vi "Variable Tool Setup GUI.vi"(11 "error in (no error)":errorcluster) -> (8 "OK":bool, 15 "error out":errorcluster)   [LabVIEW 2011]
uses:
  Measurments Handling/Update frequensies.ctl
  Measurments Handling/Scaling.ctl
  Measurments Handling/Alarm Setup Analog.ctl
  Measurments Handling/Alarm Responce.ctl
  Measurments Handling/Action List.ctl
  Measurments Handling/Limits.ctl
  Measurments Handling/User Setting DigitalChannel.ctl
  Measurments Handling/Alarm Responce dig.ctl
  GUI/Graph/Plot selector.ctl
  Measurments Handling/User Setting Analog Channel Bg.ctl
  Modem Status/Variable List Modem Status Digital.ctl
  Modem Status/Variable List Modem Status Analog.ctl
  Tool/Variable List Tool Digital.ctl
  Tool/Variable List Tool Analog.ctl
  Measurments Handling/Common/Variable List Common Digital.ctl
  Measurments Handling/Common/Variable List Common Analog.ctl
  emi Lib/Basic/0 - General/App/emi_Application Folder.vi
panel:
  in  "Tab Control":enum32{"Analog", "Digital / Status"}(tab)
  in  "Unit":u16(ring) items=["g"]
  in  "Calibrate":bool
  in  "User graph selection":bool
  in  "List of Analog variables":i32(listbox)
  out "Name":string
  out "Description":string
  out "Validity":T1
  in  "Scaling":T2={"Gain"=1.0, "Offset"=0.0} {"Offset" format="%.5f"; "Gain" format="%.5f"}
  in  "Limits and responses":T3={"Technical Error(NA)"={"Action"=enum."No Action", "Alarm"=FALSE}, "LL"={"Action"=enum."No Action", "Alarm"=FALSE}, "L"={"Action"=enum."No Action", "Alarm"=FALSE}, "H"={"Action"=enum."No Action", "Alarm"=FALSE}, "HH"={"Action"=enum."No Action", "Alarm"=FALSE}, "Limits"={"LL"=-inf, "L"=-inf, "H"=inf, "HH"=inf}} {"Limits"."H" format="%.3f"; "Limits"."L" format="%.3f"; "Limits"."HH" format="%.3f"; "Limits"."LL" format="%.3f"}
  in  "Upper left 1":T7 {"Line Width" items=["0", "1", "2", "3", "4", "5"]; "Var Tag" items=[""=0, "HVPSU Head Voltage(V)"=1, "HVPSU TS Voltage(V)"=2, "HVPSU Current(A)"=3, "Winch Depth(m)"=5, "Winch Line Speed(m/min)"=6, "Winch Wire Tension(kg)"=7, "Tool Max Temperature(degC)"=8, "Tool Acceleration Sum(g)"=15, "Tool Inclination(deg)"=16, "Tool Rotation(deg)"=17, "Head Voltage(V)"=27, "Stroke Extension(mm)"=38, "Stroke Force(tonne)"=41, "Stroker Upper Tension Sub(kg)"=44, "Tractor Upper Tension Sub(kg)"=48, "Tractor Lower Tension Sub(kg)"=49, "Tool (Controller) Temperature(degC)"=9, "Tool Acceleration X(g)"=12, "Tool Acceleration Y(g)"=13, "Tool Acceleration Z(g)"=14, "PSU Temp(degC)"=26, "Upper Tension Sub Temp(degC)"=30, "Tool Upper Tension Sub Raw(kg)"=31, "Lower Tension Sub Temp(degC)"=32, "Tool Lower Tension Sub Raw(kg)"=33, "Stroke In Force(tonne)"=39, "Stroke Out Force(tonne)"=40, "Stroker Pressure 1(bar)"=42, "Stroker Pressure 2(bar)"=43, "Tool Temperature sensor(degC)"=52, "Tool Motor Current(A)"=54, "TS_Signal_Quality(NA)"=58, "TS_Gain(NA)"=60, "DH_Signal_Quality(NA)"=61, "DH_Gain(NA)"=63, "Link_Status(NA)"=64, "PCP Cable Resistance(Ohm)"=4, "Tool Supply Voltage(V)"=10, "Tool (Controller) Current(A)"=11, "Tool GP Sensor 1(V)"=18, "Tool GP Sensor 2(V)"=19, "Tool (Pressure 1) Temperature(degC)"=20, "Tool Pressure 1 RAW(bar)"=21, "Tool (Pressure 2) Temperature(degC)"=22, "Tool Pressure 2 RAW(bar)"=23, "Tool (Solenoid) Temperature(degC)"=24, "Tool Solenoid Position(m)"=25, "PSU Main Voltage out(V)"=28, "PSU Main Current out(A)"=29, "Tool Motor Voltage(V)"=53, "Tool Motor Torque(tonne)"=55, "Tool weight on bit(tonne)"=56, "Tool Motor RPM(RPM)"=57, "TS_PCB_Temp(degC)"=59, "DH_PCB_Temp(degC)"=62]}
  in  "Upper left 2":T7 caption="Upper left 1" {"Line Width" items=["0", "1", "2", "3", "4", "5"]; "Var Tag" items=[""=0, "HVPSU Head Voltage(V)"=1, "HVPSU TS Voltage(V)"=2, "HVPSU Current(A)"=3, "Winch Depth(m)"=5, "Winch Line Speed(m/min)"=6, "Winch Wire Tension(kg)"=7, "Tool Max Temperature(degC)"=8, "Tool Acceleration Sum(g)"=15, "Tool Inclination(deg)"=16, "Tool Rotation(deg)"=17, "Head Voltage(V)"=27, "Stroke Extension(mm)"=38, "Stroke Force(tonne)"=41, "Stroker Upper Tension Sub(kg)"=44, "Tractor Upper Tension Sub(kg)"=48, "Tractor Lower Tension Sub(kg)"=49, "Tool (Controller) Temperature(degC)"=9, "Tool Acceleration X(g)"=12, "Tool Acceleration Y(g)"=13, "Tool Acceleration Z(g)"=14, "PSU Temp(degC)"=26, "Upper Tension Sub Temp(degC)"=30, "Tool Upper Tension Sub Raw(kg)"=31, "Lower Tension Sub Temp(degC)"=32, "Tool Lower Tension Sub Raw(kg)"=33, "Stroke In Force(tonne)"=39, "Stroke Out Force(tonne)"=40, "Stroker Pressure 1(bar)"=42, "Stroker Pressure 2(bar)"=43, "Tool Temperature sensor(degC)"=52, "Tool Motor Current(A)"=54, "TS_Signal_Quality(NA)"=58, "TS_Gain(NA)"=60, "DH_Signal_Quality(NA)"=61, "DH_Gain(NA)"=63, "Link_Status(NA)"=64, "PCP Cable Resistance(Ohm)"=4, "Tool Supply Voltage(V)"=10, "Tool (Controller) Current(A)"=11, "Tool GP Sensor 1(V)"=18, "Tool GP Sensor 2(V)"=19, "Tool (Pressure 1) Temperature(degC)"=20, "Tool Pressure 1 RAW(bar)"=21, "Tool (Pressure 2) Temperature(degC)"=22, "Tool Pressure 2 RAW(bar)"=23, "Tool (Solenoid) Temperature(degC)"=24, "Tool Solenoid Position(m)"=25, "PSU Main Voltage out(V)"=28, "PSU Main Current out(A)"=29, "Tool Motor Voltage(V)"=53, "Tool Motor Torque(tonne)"=55, "Tool weight on bit(tonne)"=56, "Tool Motor RPM(RPM)"=57, "TS_PCB_Temp(degC)"=59, "DH_PCB_Temp(degC)"=62]}
  in  "Upper right 1":T7 caption="Upper left 1" {"Line Width" items=["0", "1", "2", "3", "4", "5"]; "Var Tag" items=[""=0, "HVPSU Head Voltage(V)"=1, "HVPSU TS Voltage(V)"=2, "HVPSU Current(A)"=3, "Winch Depth(m)"=5, "Winch Line Speed(m/min)"=6, "Winch Wire Tension(kg)"=7, "Tool Max Temperature(degC)"=8, "Tool Acceleration Sum(g)"=15, "Tool Inclination(deg)"=16, "Tool Rotation(deg)"=17, "Head Voltage(V)"=27, "Stroke Extension(mm)"=38, "Stroke Force(tonne)"=41, "Stroker Upper Tension Sub(kg)"=44, "Tractor Upper Tension Sub(kg)"=48, "Tractor Lower Tension Sub(kg)"=49, "Tool (Controller) Temperature(degC)"=9, "Tool Acceleration X(g)"=12, "Tool Acceleration Y(g)"=13, "Tool Acceleration Z(g)"=14, "PSU Temp(degC)"=26, "Upper Tension Sub Temp(degC)"=30, "Tool Upper Tension Sub Raw(kg)"=31, "Lower Tension Sub Temp(degC)"=32, "Tool Lower Tension Sub Raw(kg)"=33, "Stroke In Force(tonne)"=39, "Stroke Out Force(tonne)"=40, "Stroker Pressure 1(bar)"=42, "Stroker Pressure 2(bar)"=43, "Tool Temperature sensor(degC)"=52, "Tool Motor Current(A)"=54, "TS_Signal_Quality(NA)"=58, "TS_Gain(NA)"=60, "DH_Signal_Quality(NA)"=61, "DH_Gain(NA)"=63, "Link_Status(NA)"=64, "PCP Cable Resistance(Ohm)"=4, "Tool Supply Voltage(V)"=10, "Tool (Controller) Current(A)"=11, "Tool GP Sensor 1(V)"=18, "Tool GP Sensor 2(V)"=19, "Tool (Pressure 1) Temperature(degC)"=20, "Tool Pressure 1 RAW(bar)"=21, "Tool (Pressure 2) Temperature(degC)"=22, "Tool Pressure 2 RAW(bar)"=23, "Tool (Solenoid) Temperature(degC)"=24, "Tool Solenoid Position(m)"=25, "PSU Main Voltage out(V)"=28, "PSU Main Current out(A)"=29, "Tool Motor Voltage(V)"=53, "Tool Motor Torque(tonne)"=55, "Tool weight on bit(tonne)"=56, "Tool Motor RPM(RPM)"=57, "TS_PCB_Temp(degC)"=59, "DH_PCB_Temp(degC)"=62]}
  in  "Upper right 2":T7 caption="Upper left 1" {"Line Width" items=["0", "1", "2", "3", "4", "5"]; "Var Tag" items=[""=0, "HVPSU Head Voltage(V)"=1, "HVPSU TS Voltage(V)"=2, "HVPSU Current(A)"=3, "Winch Depth(m)"=5, "Winch Line Speed(m/min)"=6, "Winch Wire Tension(kg)"=7, "Tool Max Temperature(degC)"=8, "Tool Acceleration Sum(g)"=15, "Tool Inclination(deg)"=16, "Tool Rotation(deg)"=17, "Head Voltage(V)"=27, "Stroke Extension(mm)"=38, "Stroke Force(tonne)"=41, "Stroker Upper Tension Sub(kg)"=44, "Tractor Upper Tension Sub(kg)"=48, "Tractor Lower Tension Sub(kg)"=49, "Tool (Controller) Temperature(degC)"=9, "Tool Acceleration X(g)"=12, "Tool Acceleration Y(g)"=13, "Tool Acceleration Z(g)"=14, "PSU Temp(degC)"=26, "Upper Tension Sub Temp(degC)"=30, "Tool Upper Tension Sub Raw(kg)"=31, "Lower Tension Sub Temp(degC)"=32, "Tool Lower Tension Sub Raw(kg)"=33, "Stroke In Force(tonne)"=39, "Stroke Out Force(tonne)"=40, "Stroker Pressure 1(bar)"=42, "Stroker Pressure 2(bar)"=43, "Tool Temperature sensor(degC)"=52, "Tool Motor Current(A)"=54, "TS_Signal_Quality(NA)"=58, "TS_Gain(NA)"=60, "DH_Signal_Quality(NA)"=61, "DH_Gain(NA)"=63, "Link_Status(NA)"=64, "PCP Cable Resistance(Ohm)"=4, "Tool Supply Voltage(V)"=10, "Tool (Controller) Current(A)"=11, "Tool GP Sensor 1(V)"=18, "Tool GP Sensor 2(V)"=19, "Tool (Pressure 1) Temperature(degC)"=20, "Tool Pressure 1 RAW(bar)"=21, "Tool (Pressure 2) Temperature(degC)"=22, "Tool Pressure 2 RAW(bar)"=23, "Tool (Solenoid) Temperature(degC)"=24, "Tool Solenoid Position(m)"=25, "PSU Main Voltage out(V)"=28, "PSU Main Current out(A)"=29, "Tool Motor Voltage(V)"=53, "Tool Motor Torque(tonne)"=55, "Tool weight on bit(tonne)"=56, "Tool Motor RPM(RPM)"=57, "TS_PCB_Temp(degC)"=59, "DH_PCB_Temp(degC)"=62]}
  in  "Lower left 1":T7 caption="Upper left 1" {"Line Width" items=["0", "1", "2", "3", "4", "5"]; "Var Tag" items=[""=0, "HVPSU Head Voltage(V)"=1, "HVPSU TS Voltage(V)"=2, "HVPSU Current(A)"=3, "Winch Depth(m)"=5, "Winch Line Speed(m/min)"=6, "Winch Wire Tension(kg)"=7, "Tool Max Temperature(degC)"=8, "Tool Acceleration Sum(g)"=15, "Tool Inclination(deg)"=16, "Tool Rotation(deg)"=17, "Head Voltage(V)"=27, "Stroke Extension(mm)"=38, "Stroke Force(tonne)"=41, "Stroker Upper Tension Sub(kg)"=44, "Tractor Upper Tension Sub(kg)"=48, "Tractor Lower Tension Sub(kg)"=49, "Tool (Controller) Temperature(degC)"=9, "Tool Acceleration X(g)"=12, "Tool Acceleration Y(g)"=13, "Tool Acceleration Z(g)"=14, "PSU Temp(degC)"=26, "Upper Tension Sub Temp(degC)"=30, "Tool Upper Tension Sub Raw(kg)"=31, "Lower Tension Sub Temp(degC)"=32, "Tool Lower Tension Sub Raw(kg)"=33, "Stroke In Force(tonne)"=39, "Stroke Out Force(tonne)"=40, "Stroker Pressure 1(bar)"=42, "Stroker Pressure 2(bar)"=43, "Tool Temperature sensor(degC)"=52, "Tool Motor Current(A)"=54, "TS_Signal_Quality(NA)"=58, "TS_Gain(NA)"=60, "DH_Signal_Quality(NA)"=61, "DH_Gain(NA)"=63, "Link_Status(NA)"=64, "PCP Cable Resistance(Ohm)"=4, "Tool Supply Voltage(V)"=10, "Tool (Controller) Current(A)"=11, "Tool GP Sensor 1(V)"=18, "Tool GP Sensor 2(V)"=19, "Tool (Pressure 1) Temperature(degC)"=20, "Tool Pressure 1 RAW(bar)"=21, "Tool (Pressure 2) Temperature(degC)"=22, "Tool Pressure 2 RAW(bar)"=23, "Tool (Solenoid) Temperature(degC)"=24, "Tool Solenoid Position(m)"=25, "PSU Main Voltage out(V)"=28, "PSU Main Current out(A)"=29, "Tool Motor Voltage(V)"=53, "Tool Motor Torque(tonne)"=55, "Tool weight on bit(tonne)"=56, "Tool Motor RPM(RPM)"=57, "TS_PCB_Temp(degC)"=59, "DH_PCB_Temp(degC)"=62]}
  in  "Lower left 2":T7 caption="Upper left 1" {"Line Width" items=["0", "1", "2", "3", "4", "5"]; "Var Tag" items=[""=0, "HVPSU Head Voltage(V)"=1, "HVPSU TS Voltage(V)"=2, "HVPSU Current(A)"=3, "Winch Depth(m)"=5, "Winch Line Speed(m/min)"=6, "Winch Wire Tension(kg)"=7, "Tool Max Temperature(degC)"=8, "Tool Acceleration Sum(g)"=15, "Tool Inclination(deg)"=16, "Tool Rotation(deg)"=17, "Head Voltage(V)"=27, "Stroke Extension(mm)"=38, "Stroke Force(tonne)"=41, "Stroker Upper Tension Sub(kg)"=44, "Tractor Upper Tension Sub(kg)"=48, "Tractor Lower Tension Sub(kg)"=49, "Tool (Controller) Temperature(degC)"=9, "Tool Acceleration X(g)"=12, "Tool Acceleration Y(g)"=13, "Tool Acceleration Z(g)"=14, "PSU Temp(degC)"=26, "Upper Tension Sub Temp(degC)"=30, "Tool Upper Tension Sub Raw(kg)"=31, "Lower Tension Sub Temp(degC)"=32, "Tool Lower Tension Sub Raw(kg)"=33, "Stroke In Force(tonne)"=39, "Stroke Out Force(tonne)"=40, "Stroker Pressure 1(bar)"=42, "Stroker Pressure 2(bar)"=43, "Tool Temperature sensor(degC)"=52, "Tool Motor Current(A)"=54, "TS_Signal_Quality(NA)"=58, "TS_Gain(NA)"=60, "DH_Signal_Quality(NA)"=61, "DH_Gain(NA)"=63, "Link_Status(NA)"=64, "PCP Cable Resistance(Ohm)"=4, "Tool Supply Voltage(V)"=10, "Tool (Controller) Current(A)"=11, "Tool GP Sensor 1(V)"=18, "Tool GP Sensor 2(V)"=19, "Tool (Pressure 1) Temperature(degC)"=20, "Tool Pressure 1 RAW(bar)"=21, "Tool (Pressure 2) Temperature(degC)"=22, "Tool Pressure 2 RAW(bar)"=23, "Tool (Solenoid) Temperature(degC)"=24, "Tool Solenoid Position(m)"=25, "PSU Main Voltage out(V)"=28, "PSU Main Current out(A)"=29, "Tool Motor Voltage(V)"=53, "Tool Motor Torque(tonne)"=55, "Tool weight on bit(tonne)"=56, "Tool Motor RPM(RPM)"=57, "TS_PCB_Temp(degC)"=59, "DH_PCB_Temp(degC)"=62]}
  in  "Lower right 1":T7 caption="Upper left 1" {"Line Width" items=["0", "1", "2", "3", "4", "5"]; "Var Tag" items=[""=0, "HVPSU Head Voltage(V)"=1, "HVPSU TS Voltage(V)"=2, "HVPSU Current(A)"=3, "Winch Depth(m)"=5, "Winch Line Speed(m/min)"=6, "Winch Wire Tension(kg)"=7, "Tool Max Temperature(degC)"=8, "Tool Acceleration Sum(g)"=15, "Tool Inclination(deg)"=16, "Tool Rotation(deg)"=17, "Head Voltage(V)"=27, "Stroke Extension(mm)"=38, "Stroke Force(tonne)"=41, "Stroker Upper Tension Sub(kg)"=44, "Tractor Upper Tension Sub(kg)"=48, "Tractor Lower Tension Sub(kg)"=49, "Tool (Controller) Temperature(degC)"=9, "Tool Acceleration X(g)"=12, "Tool Acceleration Y(g)"=13, "Tool Acceleration Z(g)"=14, "PSU Temp(degC)"=26, "Upper Tension Sub Temp(degC)"=30, "Tool Upper Tension Sub Raw(kg)"=31, "Lower Tension Sub Temp(degC)"=32, "Tool Lower Tension Sub Raw(kg)"=33, "Stroke In Force(tonne)"=39, "Stroke Out Force(tonne)"=40, "Stroker Pressure 1(bar)"=42, "Stroker Pressure 2(bar)"=43, "Tool Temperature sensor(degC)"=52, "Tool Motor Current(A)"=54, "TS_Signal_Quality(NA)"=58, "TS_Gain(NA)"=60, "DH_Signal_Quality(NA)"=61, "DH_Gain(NA)"=63, "Link_Status(NA)"=64, "PCP Cable Resistance(Ohm)"=4, "Tool Supply Voltage(V)"=10, "Tool (Controller) Current(A)"=11, "Tool GP Sensor 1(V)"=18, "Tool GP Sensor 2(V)"=19, "Tool (Pressure 1) Temperature(degC)"=20, "Tool Pressure 1 RAW(bar)"=21, "Tool (Pressure 2) Temperature(degC)"=22, "Tool Pressure 2 RAW(bar)"=23, "Tool (Solenoid) Temperature(degC)"=24, "Tool Solenoid Position(m)"=25, "PSU Main Voltage out(V)"=28, "PSU Main Current out(A)"=29, "Tool Motor Voltage(V)"=53, "Tool Motor Torque(tonne)"=55, "Tool weight on bit(tonne)"=56, "Tool Motor RPM(RPM)"=57, "TS_PCB_Temp(degC)"=59, "DH_PCB_Temp(degC)"=62]}
  in  "Lower right 2":T7 caption="Upper left 1" {"Line Width" items=["0", "1", "2", "3", "4", "5"]; "Var Tag" items=[""=0, "HVPSU Head Voltage(V)"=1, "HVPSU TS Voltage(V)"=2, "HVPSU Current(A)"=3, "Winch Depth(m)"=5, "Winch Line Speed(m/min)"=6, "Winch Wire Tension(kg)"=7, "Tool Max Temperature(degC)"=8, "Tool Acceleration Sum(g)"=15, "Tool Inclination(deg)"=16, "Tool Rotation(deg)"=17, "Head Voltage(V)"=27, "Stroke Extension(mm)"=38, "Stroke Force(tonne)"=41, "Stroker Upper Tension Sub(kg)"=44, "Tractor Upper Tension Sub(kg)"=48, "Tractor Lower Tension Sub(kg)"=49, "Tool (Controller) Temperature(degC)"=9, "Tool Acceleration X(g)"=12, "Tool Acceleration Y(g)"=13, "Tool Acceleration Z(g)"=14, "PSU Temp(degC)"=26, "Upper Tension Sub Temp(degC)"=30, "Tool Upper Tension Sub Raw(kg)"=31, "Lower Tension Sub Temp(degC)"=32, "Tool Lower Tension Sub Raw(kg)"=33, "Stroke In Force(tonne)"=39, "Stroke Out Force(tonne)"=40, "Stroker Pressure 1(bar)"=42, "Stroker Pressure 2(bar)"=43, "Tool Temperature sensor(degC)"=52, "Tool Motor Current(A)"=54, "TS_Signal_Quality(NA)"=58, "TS_Gain(NA)"=60, "DH_Signal_Quality(NA)"=61, "DH_Gain(NA)"=63, "Link_Status(NA)"=64, "PCP Cable Resistance(Ohm)"=4, "Tool Supply Voltage(V)"=10, "Tool (Controller) Current(A)"=11, "Tool GP Sensor 1(V)"=18, "Tool GP Sensor 2(V)"=19, "Tool (Pressure 1) Temperature(degC)"=20, "Tool Pressure 1 RAW(bar)"=21, "Tool (Pressure 2) Temperature(degC)"=22, "Tool Pressure 2 RAW(bar)"=23, "Tool (Solenoid) Temperature(degC)"=24, "Tool Solenoid Position(m)"=25, "PSU Main Voltage out(V)"=28, "PSU Main Current out(A)"=29, "Tool Motor Voltage(V)"=53, "Tool Motor Torque(tonne)"=55, "Tool weight on bit(tonne)"=56, "Tool Motor RPM(RPM)"=57, "TS_PCB_Temp(degC)"=59, "DH_PCB_Temp(degC)"=62]}
  out "Name Dig":string
  out "NA Indicatino":string caption="NA"
  out "Description Dig":string caption="Description"
  out "Validity Dig":T1 caption="Validity"
  out "On indication":string caption="ON / TRUE"
  out "Off Indication":string caption="OFF / FALSE"
  in  "User settings":T8
  in  "List of Digital variables":i32(listbox)
  out "Mode":bool
  in  "Help":bool
  in  "Cancel":bool
  in  "OK":bool
  # "Tab header s can be changed as wanted\n\nCustom can be used for completly ccutom behavior,\nmust then highjack  an other hidden page, for settings"
  # "Add custom behavior taht cvan not be replicated by a simple cluster with valisdity checking"
  # "Information"
  # "Usage"
  # "Chart default IO channels"
  # "Information"
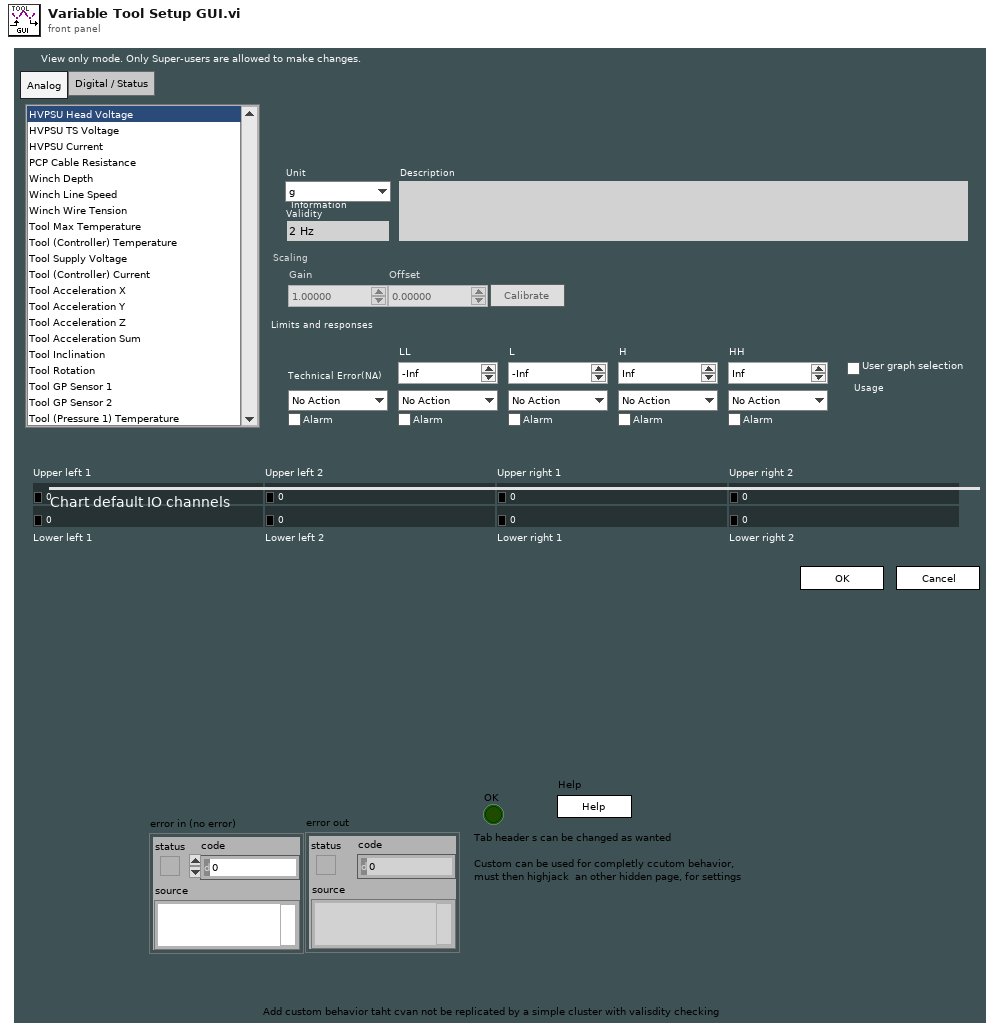
[diagram p1: front panel]
types:
  T1 = typedef "Update frequensies.ctl" = enum16{"2 Hz", "1 Hz", "0.1 Hz"}
  T2 = typedef "Scaling.ctl" = cluster{"Gain":dbl, "Offset":dbl}
  T3 = typedef "Alarm Setup Analog.ctl" = cluster{"Technical Error(NA)":T4, "LL":T4, "L":T4, "H":T4, "HH":T4, "Limits":T6}
  T4 = typedef "Alarm Responce.ctl" = cluster{"Action":T5, "Alarm":bool}
  T5 = typedef "Action List.ctl" = enum16{"No Action", "Stop Motor", "Turn Off HV"}
  T6 = typedef "Limits.ctl" = cluster{"LL":dbl, "L":dbl, "H":dbl, "HH":dbl}
  T7 = typedef "Plot selector.ctl" = cluster{"Var Tag":u16, "Color":u32, "Line Width":u16}
  T8 = typedef "User Setting DigitalChannel.ctl" = cluster{"Responses":cluster{"Technical Error (NA)":T4, "OFF / FALSE":T9, "ON / TRUE":T9}}
  T9 = typedef "Alarm Responce dig.ctl" = cluster{"Action":T5, "Alarm":bool, "Exclamation":bool}
  T10 = enum16{"GET", "SET", "Get from Ini", "Put in Ini"}
  T11 = typedef "User Indikator.ctl" = cluster{"User Name":string, "Super User":T12}
  T12 = typedef "Super User bool indikator.ctl" = bool
  T13 = enum8{"Enabled", "Disabled", "Disabled and Grayed Out"}
  T14 = typedef "Graph default cluseter.ctl" = cluster{"UL1":T7, "UL2":T7, "UR1":T7, "UR2":T7, "LL1":T7, "LL2":T7, "LR1":T7, "LR2":T7}
  T15 = typedef "Fixed Analog Channel Definition.ctl" = cluster{"ID":u16, "Name":string, "Quantity":T16, "Unit":string, "Maximum upd":T1, "Comment":string, "Help file Name":string, "Help file Section ":string, "Category":T17, "User adjustable Scaling":bool, "Default Scaling":T2, "Default Unit":i32, "Classification":T18}
  T16 = typedef "Quantity enum.ctl" = enum16{"NA", "Acceleration", "Angle", "Current", "Force", "Distance", "Pressure", "Resistance", "Rotational Speed", "Speed", "Temperature", "Tension", "Torque", "Voltage", "Weight"}
  T17 = typedef "Channel catagory Enum.ctl" = enum16{"No Category", "Power", "Temperature", "Pressure"}
  T18 = typedef "Channel Classification Enum.ctl" = enum16{"Basic", "Advanced", "Expert", "Unused"}
  T19 = typedef "Fixed Digital Channel Definition.ctl" = cluster{"ID":u16, "Name":string, "NA Text":string, "Off Text":string, "On Text":string, "Maximum upd":T1, "Comment":string, "Help file Name":string, "Help file Section ":string, "Catagory":T17, "In use":bool}
  T20 = typedef "User Setting Analog Channel Bg.ctl" = cluster{"Scaling":T2, "Limits and responces":T3, "Allow Graph selection by user":bool, "Unit":u16}
  T21 = typedef "Variable List Modem Status Digital.ctl" = enum16{"TMU_LINK_STATUS"}
  T22 = typedef "Variable List Modem Status Analog.ctl" = enum16{"TS_Signal_Quality", "TS_PCB_Temp", "TS_Gain", "DH_Signal_Quality", "DH_PCB_Temp", "DH_Gain", "Link_Status"}
  T23 = typedef "Variable List Tool Digital.ctl" = enum16{"Tool Error Controller", "Tool Stopped Controller", "Tool Relay 1", "Tool Relay 2", "Tool Both Relays", "Tool node Pressure 1", "Tool Error Pressure 1", "Tool Stopped Pressure 1", "Tool node Pressure 2", "Tool Error Pressure 2", "Tool Stopped Pressure 2", "Tool node Solenoid", "Tool Error Solenoid", "Tool Stopped Solenoid", "Tool Solenoid 1", "Tool Solenoid 2", "Tool Solenoid 3", "Tool node PSU", "Tool Error PSU", "Tool Stopped PSU", "Upper Tension Sub", "Tool Error Upper Tension Sub", "Tool Stopped Upper Tension Sub", "Lower Tension Sub", "Tool Error Lower Tension Sub", "Tool Stopped Lower Tension Sub", "Stroke Target seeking", "Stroke Moving Out", "Stroke Moving Inn", "Stroke valves set for Out", "Stroke valves set for In", "Stroke In (force)", "Stroke Out (force)", "Stroke Force decreasing(in)", "Stroke Force decreasing(out)", "Stroke Force change not correct", "Stroke SLIPS established P1", "Stroke SLIPS established P2", "Stroke SLIPS established", "Stroke Pressure Monitor Ongoing", "Stroke Pressure Monitor Ending ", "Tool Stroke enable Valve", "Tool Stroke direction Valve", "Tool Anchor Valve", "Stroker Var19 - Reserved", "Stroker Var20 - Reserved", "Stroker Var21 - Reserved", "Stroker Var22 - Reserved", "Stroker Var23 - Reserved", "Stroker Var24 - Reserved", "Tractor Var1 - Reserved", "Tractor Var2 - Reserved", "Tractor Var3 - Reserved", "Tractor Var4 - Reserved", "Tractor Var5 - Reserved", "Tractor Var6 - Reserved", "Tractor Var7 - Reserved", "Tractor Var8 - Reserved", "Oil filling mode", "Mill Bit Direction", "Position control", "Anchor", "Driller Var5 - Reserved", "Driller Var6 - Reserved", "Driller Var7 - Reserved", "Driller Var8 - Reserved"}
  T24 = typedef "Variable List Tool Analog.ctl" = enum16{"Tool Max Temperature", "Tool (Controller) Temperature", "Tool Supply Voltage", "Tool (Controller) Current", "Tool Acceleration X", "Tool Acceleration Y", "Tool Acceleration Z", "Tool Acceleration Sum", "Tool Inclination", "Tool Rotation", "Tool GP Sensor 1", "Tool GP Sensor 2", "Tool (Pressure 1) Temperature", "Tool Pressure 1 RAW", "Tool (Pressure 2) Temperature", "Tool Pressure 2 RAW", "Tool (Solenoid) Temperature", "Tool Solenoid Position", "PSU Temp", "Head Voltage", "PSU Main Voltage out", "PSU Main Current out", "Upper Tension Sub Temp", "Tool Upper Tension Sub Raw", "Lower Tension Sub Temp", "Tool Lower Tension Sub Raw", "Tool Var27 - Reserved", "Tool Var28 - Reserved", "Tool Var29 - Reserved", "Tool Var30 - Reserved", "Stroke Extension", "Stroke In Force", "Stroke Out Force", "Stroke Force", "Stroker Pressure 1", "Stroker Pressure 2", "Stroker Upper Tension Sub", "Stroker Lower Tension Sub", "Stroker Var09 - Reserved", "Stroker Var10 - Reserved", "Tractor Upper Tension Sub", "Tractor Lower Tension Sub", "Tractor Var03 - Reserved", "Tractor Var04 - Reserved", "Tool Temperature sensor", "Tool Motor Voltage", "Tool Motor Current", "Tool Motor Torque", "Tool weight on bit", "Tool Motor RPM"}
  T25 = typedef "Variable List Common Digital.ctl" = enum16{"PCP Connected", "PCP PC Control", "HV PSU connected", "HV PSU HV Active", "Modem Connected", "Tool Connected", "CanBus interface"}
  T26 = typedef "Variable List Common Analog.ctl" = enum16{"HVPSU Head Voltage", "HVPSU TS Voltage", "HVPSU Current", "PCP Cable Resistance", "Winch Depth", "Winch Line Speed", "Winch Wire Tension"}
  T27 = cluster{"Keep":bool, "Zero":bool, "2 point":bool}
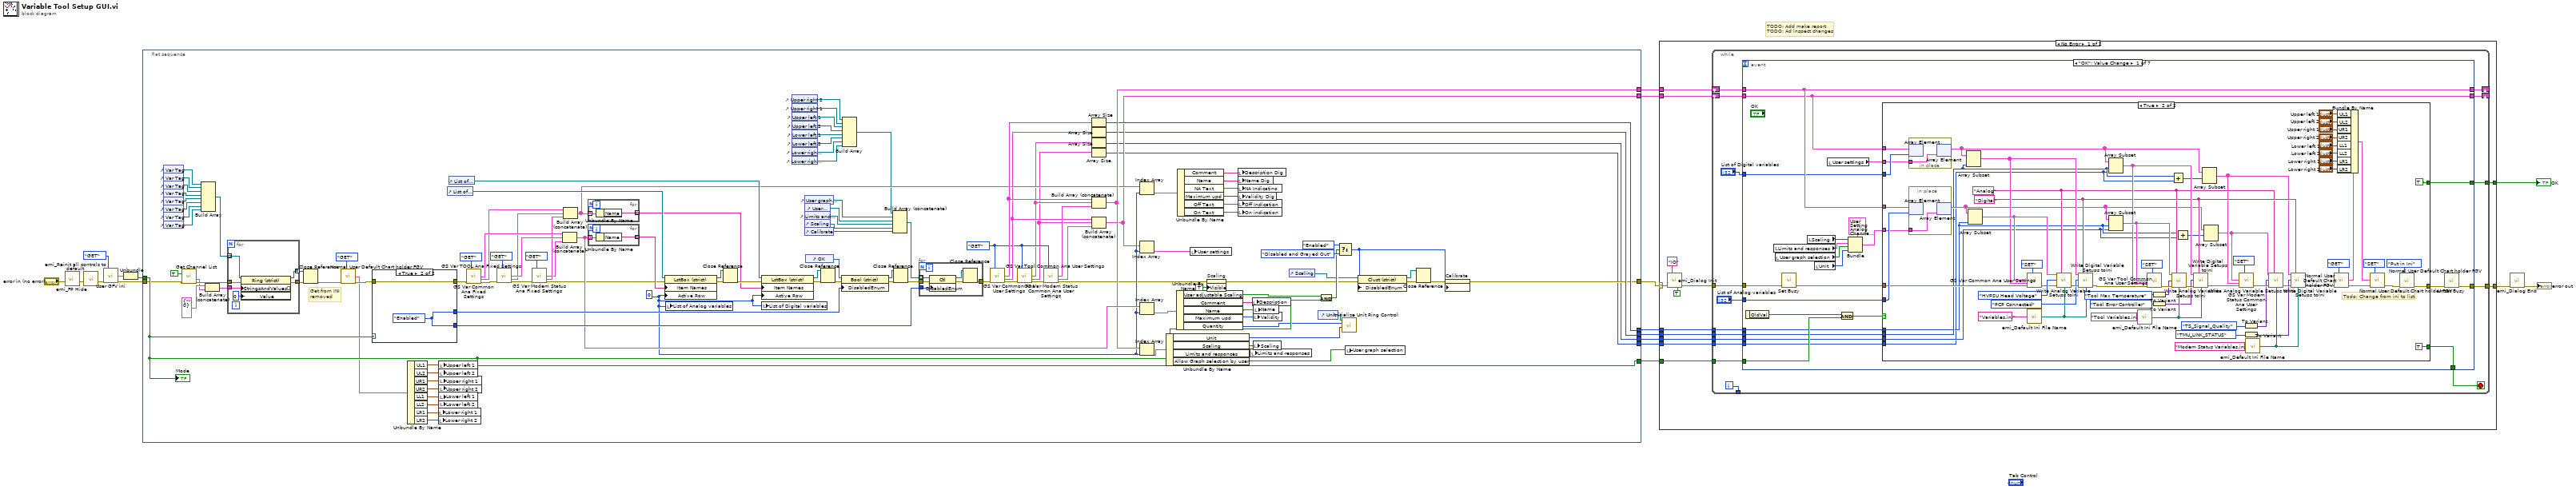
[diagram p0: block diagram]
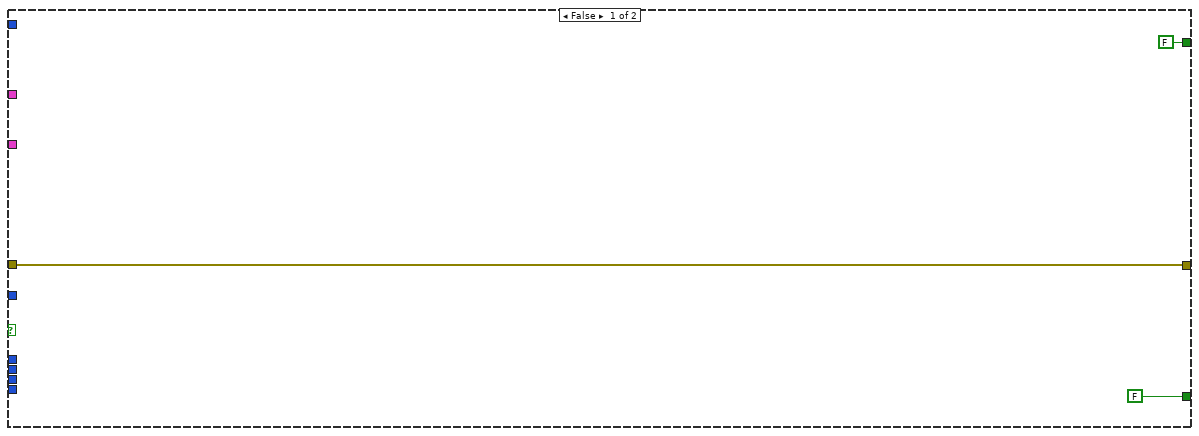
[diagram p2: hidden frame]
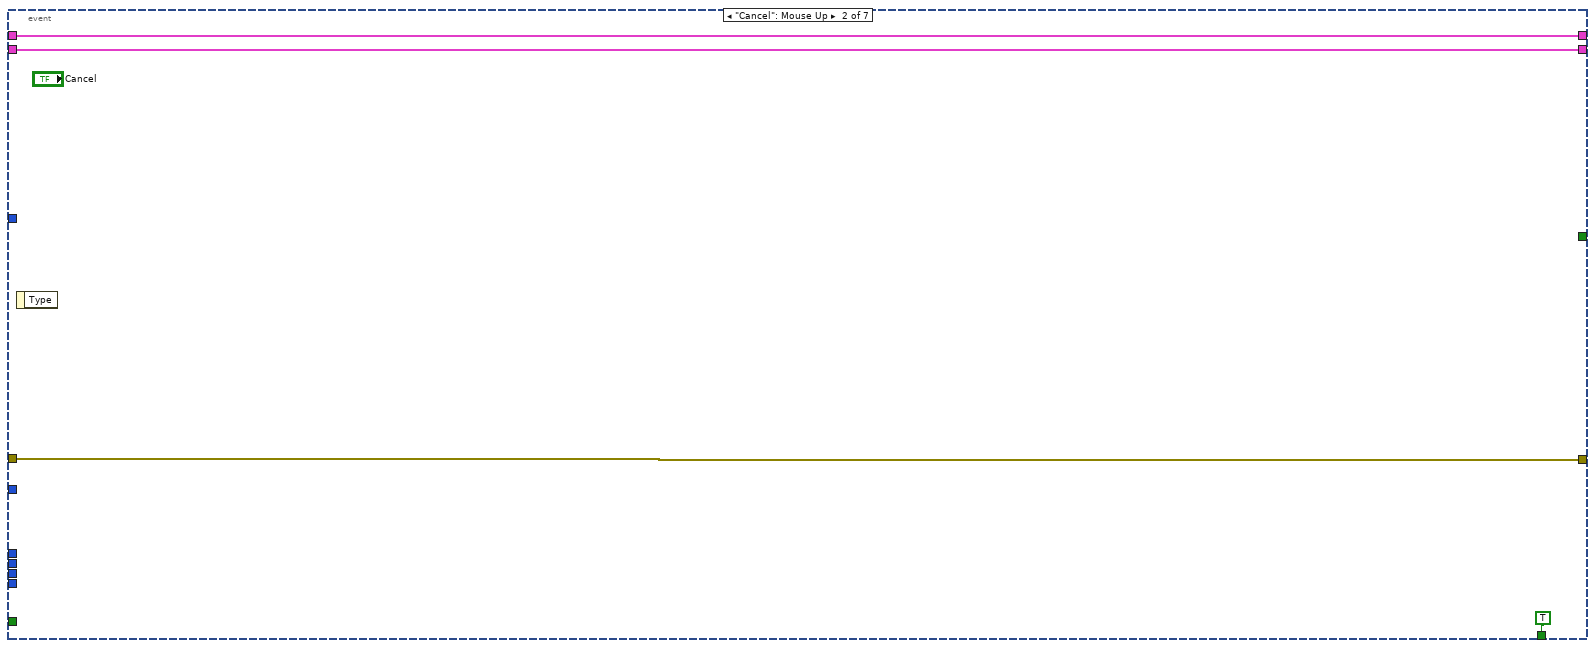
[diagram p3: hidden frame]
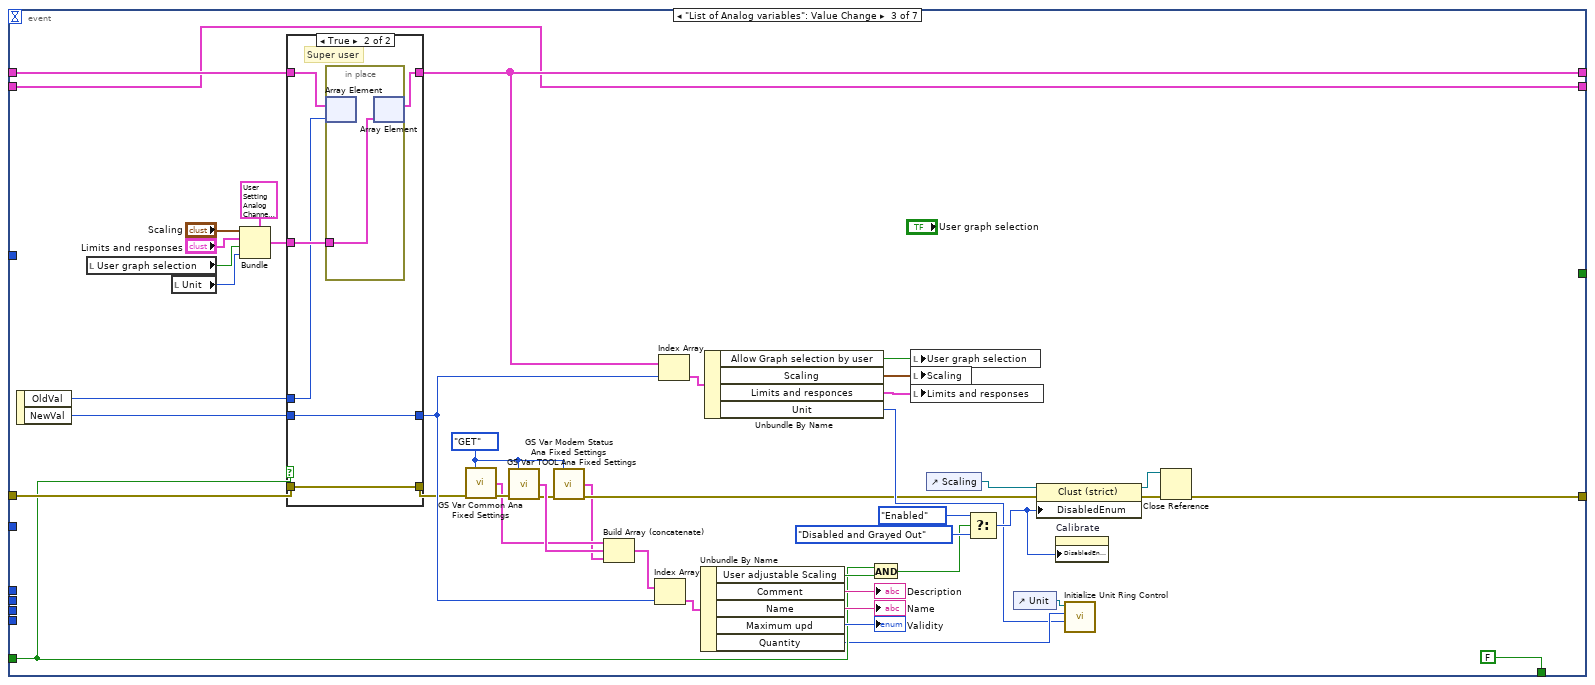
[diagram p4: hidden frame]
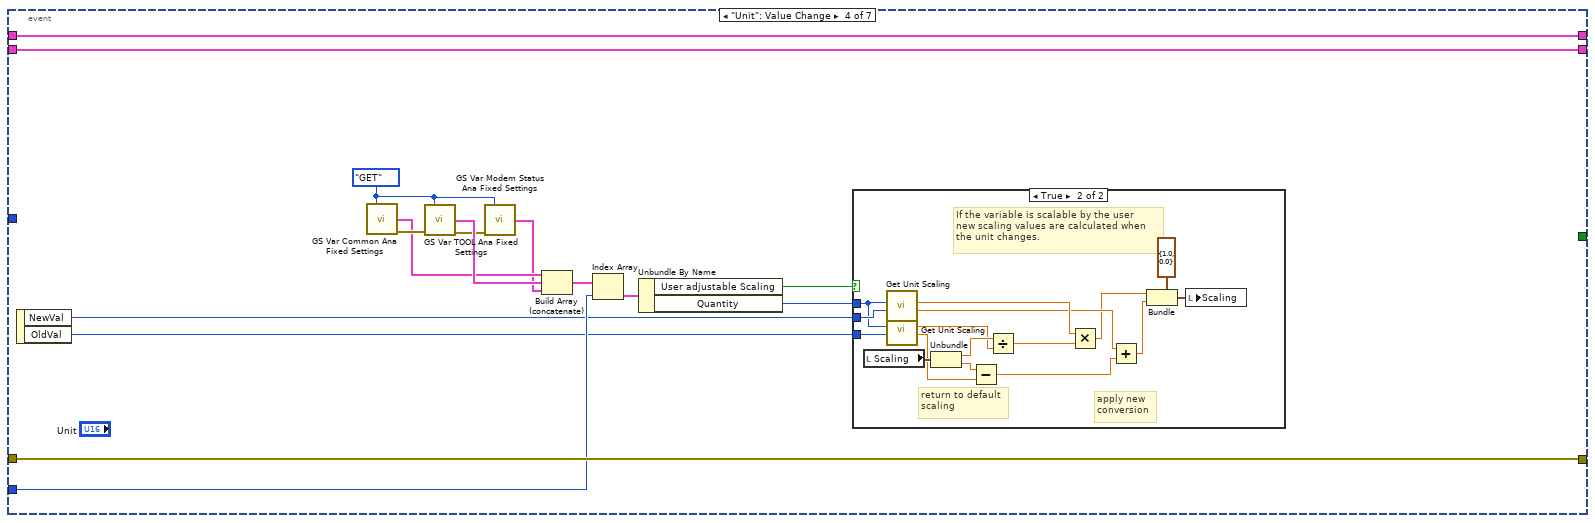
[diagram p6: hidden frame]
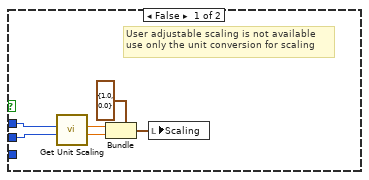
[diagram p7: hidden frame]
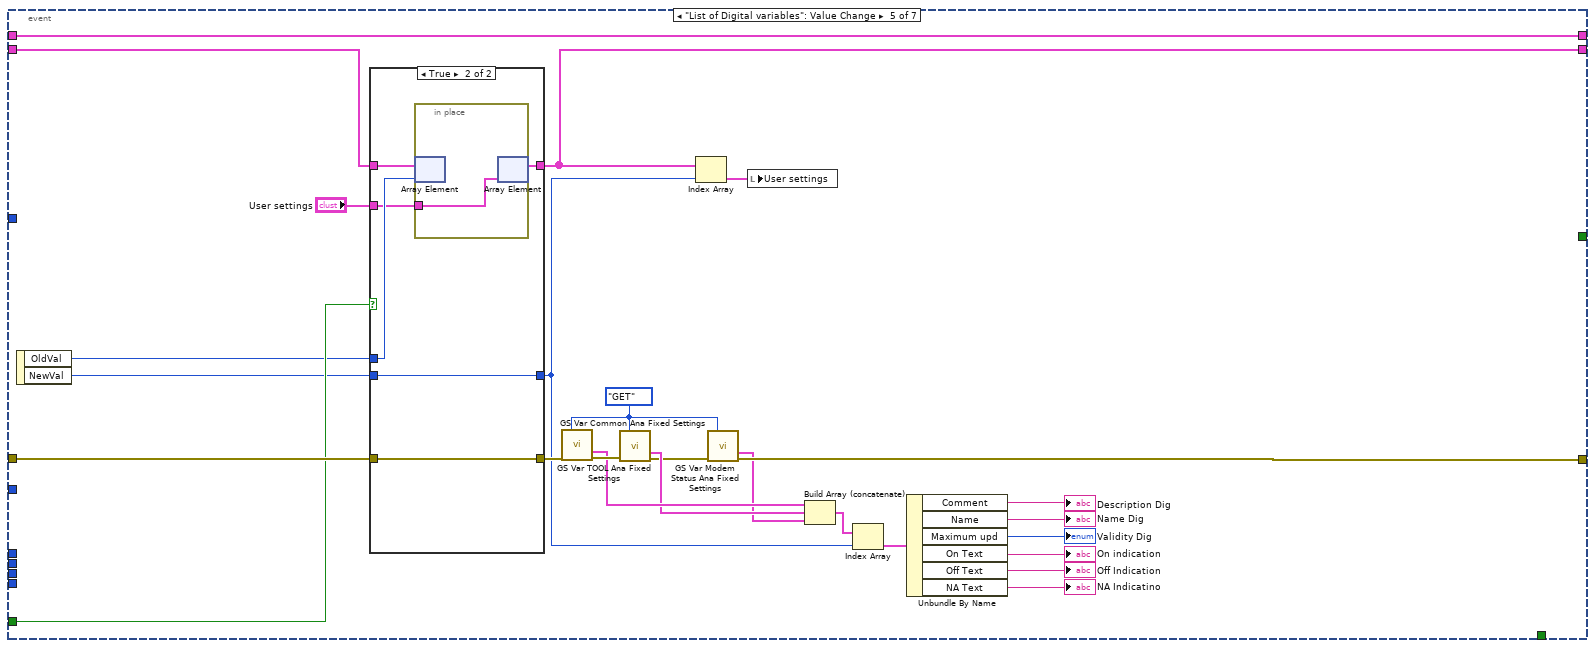
[diagram p8: hidden frame]
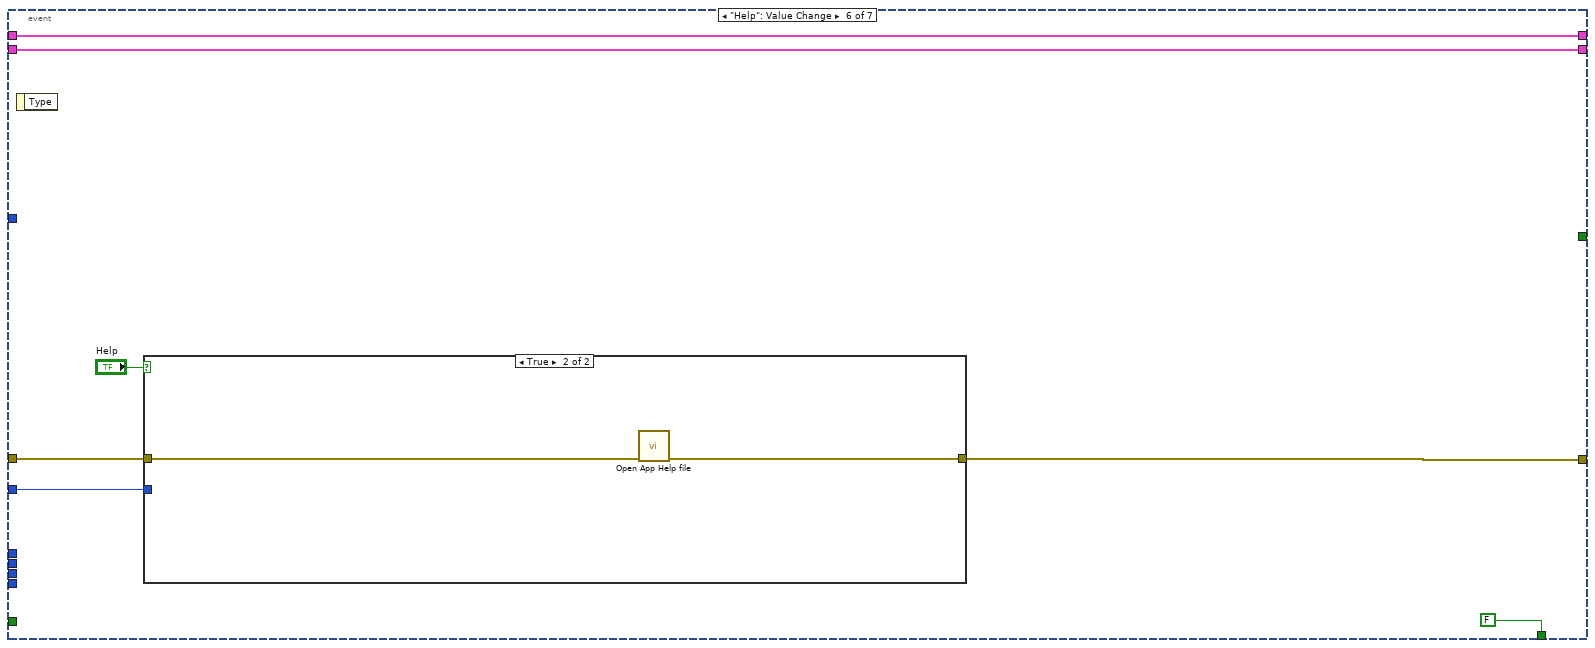
[diagram p10: hidden frame]
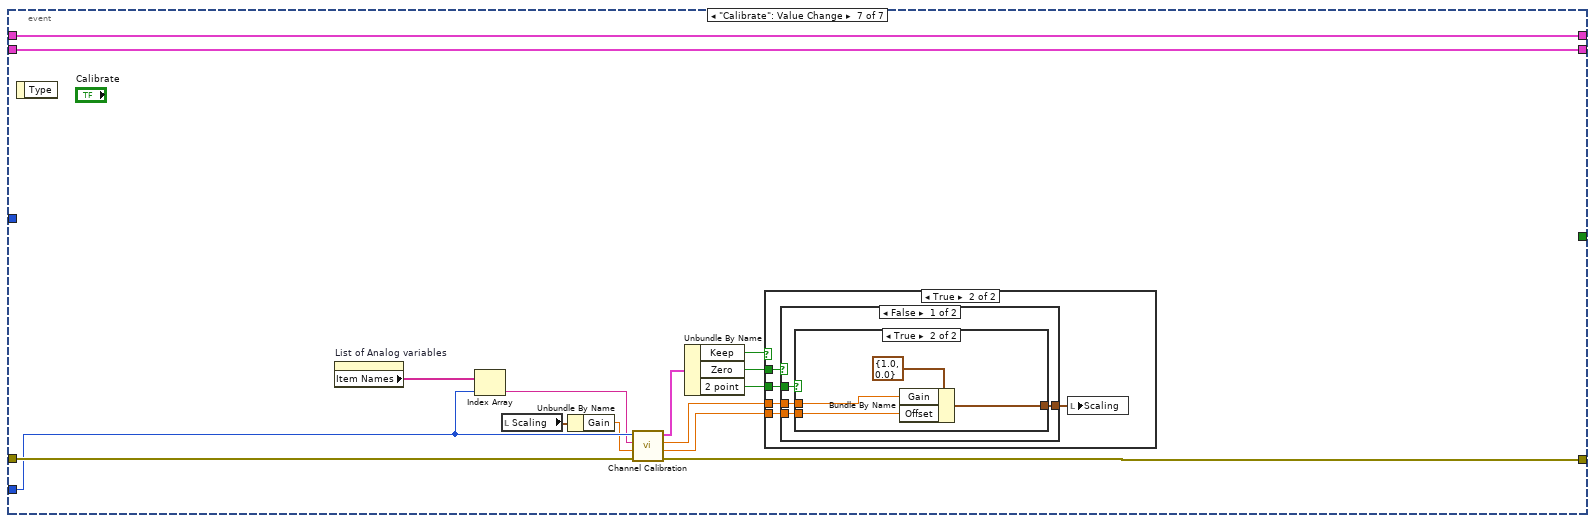
[diagram p12: hidden frame]
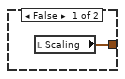
[diagram p14: hidden frame]
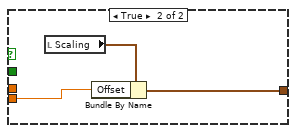
[diagram p15: hidden frame]
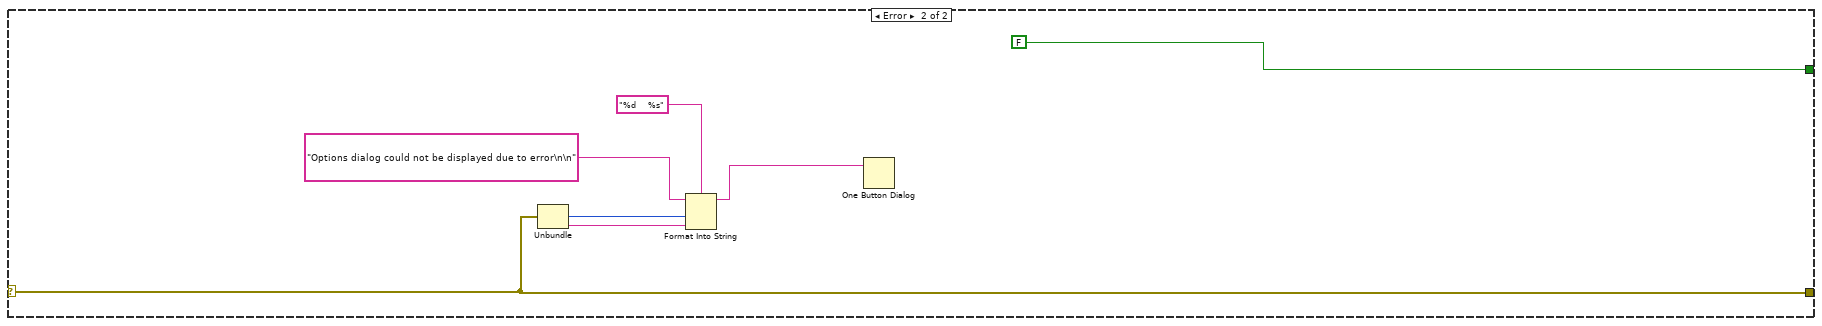
[diagram p16: hidden frame]
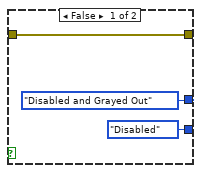
[diagram p17: hidden frame]
diagram:
  # "TODO: Add make report\nTODO: Ad inspect changes"
  n1 = call "emi_FP Hide.vi"("error in (no error)"="error in (no error)") -> ("error out"=w14:errorcluster)  [unwired: 13 in, 1 out]
  n2 = call "emi_Reinit all controls to default.vi"("error in (no error)"=w14) -> ("error out"=w12:errorcluster)  [unwired: 13 in, 1 out]
  n3 = call "User GFV ini.vi"("Action(GET)"=T10."GET", "error in (no error)"=w12) -> ("User ID out"=w11:T11, "error out"=w10:errorcluster)  [unwired: 12 in]
  n4 = Unbundle(w11) -> ("Super User"=w9:T12)  [unwired: 1 out]
  n5 = flat-sequence {
    tunnel: [w45] -> w13
    tunnel: w10 -> [w61]
    tunnel: w9 -> [w87]
    tunnel: [w87] -> w8
    tunnel: [w124] -> w7
    tunnel: [w122] -> w5
    tunnel: [w91] -> w4
    tunnel: [w90] -> w3
    tunnel: [w21] -> w2
    tunnel: [w20] -> w1
    frame #0 {
      w26 = enum16{"GET", "SET"}."GET" ("Action(GET)")
      w93 = 0 ("Active Row:Active Row Number")
      # "Get from INI\nremoved"
      n6 = control-ref of="Var Tag"() -> (w78:refnum<vi>)
      n7 = control-ref of="Var Tag"() -> (w79:refnum<vi>)
      n8 = control-ref of="Var Tag"() -> (w80:refnum<vi>)
      n9 = control-ref of="Var Tag"() -> (w81:refnum<vi>)
      n10 = control-ref of="Var Tag"() -> (w82:refnum<vi>)
      n11 = control-ref of="Var Tag"() -> (w83:refnum<vi>)
      n12 = control-ref of="Var Tag"() -> (w84:refnum<vi>)
      n13 = control-ref of="Var Tag"() -> (w85:refnum<vi>)
      n14 = call "Get Channel List.vi"("Force all(F)"=TRUE, "error in"=w61) -> ("Ring list"=w71:cluster{"String":string, "Value":u16}[], "error out"=w76:errorcluster)  [unwired: 9 in, 3 out]
      n15 = Build Array(w78, w79, w80, w81, w82, w83, w84, w85) -> (w86:refnum<vi>[])
      n16 = Build Array (concatenate)(cluster{"String":string, "Value":i32} {"String"="", "Value"=0}, w71) -> (w77:cluster{"String":string, "Value":i32}[])
      n17 = for {
        tunnel: w76 -> [w153]
        tunnel: w77 -> [w148]
        tunnel: w86 -> [w150] mode=indexing
        tunnel: [w152] -> w74
        tunnel: [w151] -> w75 mode=indexing
        n18 = property class="Ring (strict)"(reference=w150, error in=w153, "StringsAndValues[]"=w148, "Value"=u16 0) -> (reference out=w151:refnum<vi>, error out=w152:errorcluster)
      }
      n19 = Close Reference(reference=w75, error in (no error)=w74) -> (error out=w19:errorcluster)
      n20 = call "Normal User Default Chart holder FGV.vi"("Action(GET)"=T10."GET", "error in (no error)"=w19) -> ("Mem Ctl Out"=w58:T14, "error out"=w60:errorcluster)  [unwired: 12 in]
      n21 = case shown="True" w87 {
        tunnel: w60 -> [w161 w164]
        tunnel: [w161 w164] -> w140
        tunnel: [T13."Disabled and Grayed Out" ("Disabled") w163] -> w128
        tunnel: [T13."Disabled" ("Disabled") w163] -> w129
        frame False {
        }
        frame True {
          w163 = T13."Enabled" ("Disabled")
        }
      }
      n22 = Unbundle By Name(w58) -> ("UL1"=w57:T7, "UL2"=w56:T7, "UR1"=w55:T7, "UR2"=w54:T7, "LL1"=w53:T7, "LL2"=w52:T7, "LR1"=w51:T7, "LR2"=w50:T7)
      n23 = local write "Lower right 1"(w51) -> ()
      n24 = local write "Lower right 2"(w50) -> ()
      n25 = local write "Upper left 1"(w57) -> ()
      n26 = local write "Upper left 2"(w56) -> ()
      n27 = local write "Upper right 1"(w55) -> ()
      n28 = local write "Upper right 2"(w54) -> ()
      n29 = local write "Lower left 1"(w53) -> ()
      n30 = local write "Lower left 2"(w52) -> ()
      n31 = control-ref of="List of Analog variables"() -> (w139:refnum<vi>)
      n32 = control-ref of="List of Digital variables"() -> (w105:refnum<vi>)
      n33 = call "GS Var Common Ana Fixed Settings.vi"("Action(GET)"=enum16{"GET", "SET"}."GET", "error in (no error)"=w140) -> ("Common Analog Var Fixed out"=w39:T15[], "Common Digital var Fixed"=w38:T19[], "error out"=w40:errorcluster)  [unwired: 11 in]
      n34 = call "GS Var TOOL Ana Fixed Settings.vi"("Action(GET)"=enum16{"GET", "SET"}."GET", "error in (no error)"=w40) -> ("Tool Analog var Fixed out"=w42:T15[], "Tool Digital Var Fixed out"=w37:T19[], "error out"=w33:errorcluster)  [unwired: 11 in]
      n35 = call "GS Var Modem Status Ana Fixed Settings.vi"("Action(GET)"=enum16{"GET", "SET"}."GET", "error in (no error)"=w33) -> ("Modem Status Analog var Fixed out"=w29:T15[], "Modem Status Digital Var Fixed out"=w30:T19[], "error out"=w32:errorcluster)  [unwired: 11 in]
      n36 = Build Array (concatenate)(w39, w42, w29) -> (w127:T15[])
      n37 = Build Array (concatenate)(w38, w37, w30) -> (w102:T19[])
      n38 = for {
        tunnel: w102 -> [w145] mode=indexing
        tunnel: [w144] -> w104 mode=indexing
        n39 = Unbundle By Name(w145) -> ("Name"=w144:string)
      }
      n40 = for {
        tunnel: w127 -> [w147] mode=indexing
        tunnel: [w146] -> w136 mode=indexing
        n41 = Unbundle By Name(w147) -> ("Name"=w146:string)
      }
      n42 = property class="LstBox (strict)"(reference=w139, error in=w32, "Item Names"=w136, "Active Row"=w93) -> (reference out=w137:refnum<vi>, error out=w138:errorcluster)
      n43 = local write "List of Analog variables"(w93) -> ()
      n44 = Close Reference(reference=w137, error in (no error)=w138) -> (error out=w107:errorcluster)
      n45 = property class="LstBox (strict)"(reference=w105, error in=w107, "Item Names"=w104, "Active Row"=w93) -> (reference out=w109:refnum<vi>, error out=w108:errorcluster)
      n46 = local write "List of Digital variables"(w93) -> ()
      n47 = control-ref of="Upper right 2"() -> (w63:refnum<vi>)
      n48 = control-ref of="Upper right 1"() -> (w64:refnum<vi>)
      n49 = control-ref of="Upper left 1"() -> (w65:refnum<vi>)
      n50 = control-ref of="Upper left 2"() -> (w66:refnum<vi>)
      n51 = control-ref of="Lower left 1"() -> (w67:refnum<vi>)
      n52 = control-ref of="Lower left 2"() -> (w68:refnum<vi>)
      n53 = control-ref of="Lower right 1"() -> (w69:refnum<vi>)
      n54 = control-ref of="Lower right 2"() -> (w70:refnum<vi>)
      n55 = control-ref of="User settings"() -> (w103:refnum<vi>)
      n56 = control-ref of="Limits and responses"() -> (w119:refnum<vi>)
      n57 = control-ref of="Scaling"() -> (w118:refnum<vi>)
      n58 = control-ref of="User graph selection"() -> (w88:refnum<vi>)
      n59 = control-ref of="Calibrate"() -> (w44:refnum<vi>)
      n60 = control-ref of="OK"() -> (w143:refnum<vi>)
      n61 = Close Reference(reference=w109, error in (no error)=w108) -> (error out=w106:errorcluster)
      n62 = property class="Bool (strict)"(reference=w143, error in=w106, "DisabledEnum"=w128) -> (reference out=w141:refnum<vi>, error out=w142:errorcluster)
      n63 = Build Array(w63, w64, w65, w66, w67, w68, w69, w70) -> (w62:refnum<vi>[])
      n64 = Build Array (concatenate)(w62, w88, w103, w119, w118, w44) -> (w117:refnum<vi>[])
      n65 = Close Reference(reference=w141, error in (no error)=w142) -> (error out=w130:errorcluster)
      n66 = for {
        tunnel: w130 -> [w157]
        tunnel: w129 -> [w156]
        tunnel: [w155] -> w126
        tunnel: w117 -> [w154] mode=indexing
        n67 = property class="Ctl"(reference=w154, error in=w157, "DisabledEnum"=w156) -> (reference out=w159:refnum<vi>, error out=w158:errorcluster)
        n68 = Close Reference(reference=w159, error in (no error)=w158) -> (error out=w155:errorcluster)
      }
      n69 = call "GS Var Common Ana User Settings.vi"("Action(GET)"=w26, "error in (no error)"=w126) -> ("Common Analog var User set out"=w123:T20[], "Common Digital Var User set out"=w94:T8[], "error out"=w125:errorcluster)  [unwired: 11 in]
      n70 = call "GS Var Tool Common Ana User Settings.vi"("Action(GET)"=w26, "error in (no error)"=w125) -> ("Tool Analog var User settigns out"=w23:T20[], "Tool digital var User settigns out"=w22:T8[], "error out"=w28:errorcluster)  [unwired: 11 in]
      n71 = call "GS Var Modem Status Common Ana User Settings.vi"("Action(GET)"=w26, "error in (no error)"=w28) -> ("Modem Status Analog var User settigns out"=w25:T20[], "Modem Status digital var User settigns out"=w24:T8[], "error out"=w27:errorcluster)  [unwired: 11 in]
      n72 = Array Size(array=w123) -> (size(s)=w122:i32)
      n73 = Array Size(array=w94) -> (size(s)=w90:i32)
      n74 = Array Size(array=w23) -> (size(s)=w21:i32)
      n75 = Array Size(array=w22) -> (size(s)=w20:i32)
      n76 = Build Array (concatenate)(w123, w23, w25) -> (w124:T20[])
      n77 = Build Array (concatenate)(w94, w22, w24) -> (w91:T8[])
      n78 = Index Array(array=w102, index=w93) -> (element=w101:T19)
      n79 = Index Array(array=w127, index=w93) -> (element=w135:T15)
      n80 = Index Array(array=w124, index=w93) -> (element=w131:T20)
      n81 = Index Array(array=w91, index=w93) -> (element=w92:T8)
      n82 = Unbundle By Name(w131) -> ("Unit"=w34:u16, "Scaling"=w121:T2, "Limits and responces"=w120:T3, "Allow Graph selection by user"=w89:bool)
      n83 = Unbundle By Name(w135) -> ("User adjustable Scaling"=w111:bool, "Comment"=w132:string, "Name"=w133:string, "Maximum upd"=w134:T1, "Quantity"=w35:T16)
      n84 = Unbundle By Name(w101) -> ("Comment"=w100:string, "Name"=w99:string, "NA Text"=w97:string, "Maximum upd"=w98:T1, "Off Text"=w96:string, "On Text"=w95:string)
      n85 = local write "User settings"(w92) -> ()
      n86 = property on="Scaling" class="Clust (strict)"(error in=w27, "Visible"=TRUE) -> (error out=w49:errorcluster)  [unwired: 1 in, 1 out]
      n87 = local write "Description Dig"(w100) -> ()
      n88 = local write "Name Dig"(w99) -> ()
      n89 = local write "NA Indicatino"(w97) -> ()
      n90 = local write "Validity Dig"(w98) -> ()
      n91 = local write "Off Indication"(w96) -> ()
      n92 = local write "On indication"(w95) -> ()
      n93 = local write "Limits and responses"(w120) -> ()
      n94 = local write "Description"(w132) -> ()
      n95 = local write "Validity"(w134) -> ()
      n96 = local write "Scaling"(w121) -> ()
      n97 = local write "Name"(w133) -> ()
      n98 = control-ref of="Scaling"() -> (w110:refnum<vi>)
      n99 = control-ref of="Unit"() -> (w36:refnum<vi>)
      n100 = And(x=w111, y=w87) -> (x .and. y?=w113:T12)
      n101 = Select(t=T13."Enabled" ("Disabled"), s=w113, f=T13."Disabled and Grayed Out" ("Disabled")) -> (s? t:f=w47:T13)
      n102 = call "Initialize Unit Ring Control.vi"("Value"=w34, "Quantity"=w35, "Ctrl Ref"=w36) -> ()  [unwired: 9 in]
      n103 = local write "User graph selection"(w89) -> ()
      n104 = property class="Clust (strict)"(reference=w110, error in=w49, "DisabledEnum"=w47) -> (reference out=w115:refnum<vi>, error out=w114:errorcluster)
      n105 = Close Reference(reference=w115, error in (no error)=w114) -> (error out=w46:errorcluster)
      n106 = property on="Calibrate" class="Bool"(error in=w46, "DisabledEnum"=w47) -> (error out=w45:errorcluster)  [unwired: 1 in, 1 out]
      "Mode" <- w87
    }
  }
  n107 = case shown="No Error" w13 {
    selector: w13 -> [w172 w471]
    tunnel: [w177 FALSE] -> w17
    tunnel: [w176 w471] -> w16
    tunnel: w8 -> [w171 _]
    tunnel: w7 -> [w170 _]
    tunnel: w5 -> [w169 _]
    tunnel: w4 -> [w168 _]
    tunnel: w3 -> [w167 _]
    tunnel: w2 -> [w166 _]
    tunnel: w1 -> [w165 _]
    frame No Error {
      n108 = call "emi_Dialog Init.vi"("Header String(\"\")"="IO" ("Header String(\"\")"), "error in"=w172, "Modal(T)"=TRUE) -> ("error out"=w175:errorcluster)  [unwired: 12 in]
      n109 = while {
        tunnel: [w193] -> _
        tunnel: w175 -> [w191]
        tunnel: [w190] -> w176
        tunnel: [w189] -> w177
        tunnel: w171 -> [w188]
        shift-right: [w186] -> _
        shift-left: w170 -> [w187]
        tunnel: w169 -> [w184]
        shift-right: [w182] -> _
        shift-left: w168 -> [w183]
        tunnel: w167 -> [w180]
        tunnel: w166 -> [w179]
        tunnel: w165 -> [w178]
        i -> [w193]
        stop <- w192 stop-if-true
        n110 = event shown="[0] \"OK\": Value Change" {
          selector: _ -> [_ _ _ _ _ _ _]
          dyn-events: _ -> [_ _ _ _ _ _ _]
          timeout: _ -> [_ _ _ _ _ _ _]
          tunnel: [w198 TRUE FALSE _ _ FALSE _] -> w192
          tunnel: w191 -> [w217 w294 w338 w365 w412 w428 w446]
          tunnel: [w211 w294 w312 w365 w390 w429 w445] -> w190
          tunnel: [w199 _ _ _ _ _ _] -> w189
          tunnel: w188 -> [w215 _ w316 _ w411 _ _]
          tunnel: w187 -> [w214 w293 w337 w355 w413 w426 w448]
          tunnel: [w214 w293 w330 w355 w413 w426 w448] -> w186
          tunnel: "List of Analog variables" -> [w213 _ _ w357 _ w425 w437]
          tunnel: w184 -> [w210 _ _ _ _ _ _]
          tunnel: w183 -> [w205 w292 w311 w364 w410 w424 w447]
          tunnel: [w205 w292 w311 w364 w394 w424 w447] -> w182
          tunnel: "List of Digital variables" -> [w204 _ _ _ _ _ _]
          tunnel: w180 -> [w202 _ _ _ _ _ _]
          tunnel: w179 -> [w195 _ _ _ _ _ _]
          tunnel: w178 -> [w194 _ _ _ _ _ _]
          event "OK": Value Change {
            n111 = event-data() -> ("OldVal"=w200:bool)  [unwired: 1 in]
            n112 = local read "Limits and responses"() -> (w209:T3)
            n113 = local read "User graph selection"() -> (w197:bool)
            n114 = call <vilib>:"Set Busy.vi"("error in (no error)"=w217) -> ("error out"=w212:errorcluster)  [unwired: 9 in, 1 out]
            n115 = local read "Scaling"() -> (w208:T2)
            n116 = local read "Unit"() -> (w196:u16)
            n117 = local read "User settings"() -> (w203:T8)
            n118 = And(x=w200, y=w215) -> (x .and. y?=w201:T12)
            n119 = Bundle(cluster=T20 {"Scaling"={"Gain"=0.0, "Offset"=0.0}, "Limits and responces"={"Technical Error(NA)"={"Action"=enum."No Action", "Alarm"=FALSE}, "LL"={"Action"=enum."No Action", "Alarm"=FALSE}, "L"={"Action"=enum."No Action", "Alarm"=FALSE}, "H"={"Action"=enum."No Action", "Alarm"=FALSE}, "HH"={"Action"=enum."No Action", "Alarm"=FALSE}, "Limits"={"LL"=0.0, "L"=0.0, "H"=0.0, "HH"=0.0}}, "Allow Graph selection by user"=FALSE, "Unit"=0} ("element"), "Scaling"=w208, "Limits and responces"=w209, "Allow Graph selection by user"=w197, "Unit"=w196) -> (w206:T20)
            n120 = case shown="True" w201 {
              tunnel: w212 -> [w220 w281]
              tunnel: [w220 w266] -> w216
              tunnel: w214 -> [_ w289]
              tunnel: w213 -> [_ w288]
              tunnel: w206 -> [_ w287]
              tunnel: w210 -> [_ w225]
              tunnel: w205 -> [_ w278]
              tunnel: w204 -> [_ w279]
              tunnel: w203 -> [_ w277]
              tunnel: w202 -> [_ w227]
              tunnel: [FALSE TRUE] -> w199
              tunnel: [FALSE TRUE] -> w198
              tunnel: w195 -> [_ w222]
              tunnel: w194 -> [_ w221]
              frame False {
              }
              frame True {
                w236 = "Digital" ("Section(\"Default\")")
                w235 = "Analog" ("Section(\"Default\")")
                # "Todo: Change from ini to list"
                n121 = in-place {
                  in-place-border: w277 -> [w290]
                  n122 = in-place-array #1(w278, w279) -> ()  [unwired: 1 out]
                  n123 = in-place-array #1(w290) -> (w223:T8[])  [unwired: 1 out]
                }
                n124 = in-place {
                  in-place-border: w287 -> [w291]
                  n125 = in-place-array #2(w289, w288) -> ()  [unwired: 1 out]
                  n126 = in-place-array #2(w291) -> (w229:T20[])  [unwired: 1 out]
                }
                n127 = Array Subset(array=w223, length=w227) -> (w271:T8[])  [unwired: 1 in]
                n128 = Array Subset(array=w229, length=w225) -> (w280:T20[])  [unwired: 1 in]
                n129 = call "GS Var Common Ana User Settings.vi"("Action(GET)"=enum16{"GET", "SET"}."SET", "Common variables User settigns in"=w280, "Common Digital Var User set in"=w271, "error in (no error)"=w281) -> ("error out"=w283:errorcluster)  [unwired: 9 in, 2 out]
                n130 = call "emi_Default Ini File Name.vi"("Name"="Variables.ini" ("name or relative path")) -> ("Path"=w250:path)  [unwired: 13 in, 1 out]
                n131 = call "Write Analog Variable Setups toIni.vi"("error in (no error)"=w283, "Path"=w250, "Enum with Variable List"=Variable_List_Common_Analog."HVPSU Head Voltage" ("Action"), "Analog User settigns"=w280, "Section(\"Default\")"=w235) -> ("error out"=w276:errorcluster)  [unwired: 10 in]
                n132 = call "Write Digital Variable Setups toIni.vi"("error in (no error)"=w276, "Path"=w250, "Enum with Variable List"=Variable_List_Common_Digital."PCP Connected" ("Action"), "Digital User settigns"=w271, "Section(\"Default\")"=w236) -> ("error out"=w274:errorcluster)  [unwired: 10 in]
                n133 = Array Subset(array=w223, index=w227, length=w221) -> (w270:T8[])
                n134 = Array Subset(array=w229, index=w225, length=w222) -> (w285:T20[])
                n135 = call "emi_Default Ini File Name.vi"("Name"="Tool Variables.ini" ("name or relative path")) -> ("Path"=w246:path)  [unwired: 13 in, 1 out]
                n136 = call "GS Var Tool Common Ana User Settings.vi"("Action(GET)"=enum16{"GET", "SET"}."SET", "Tool analog var User settigns in"=w285, "Tool digital var User settigns in"=w270, "error in (no error)"=w274) -> ("error out"=w273:errorcluster)  [unwired: 9 in, 2 out]
                n137 = To Variant(anything=Variable_List_Tool_Analog."Tool Max Temperature" ("Variable ID")) -> (Variant=w248:variant)
                n138 = To Variant(anything=Variable_List_Tool_Digital."Tool Error Controller") -> (Variant=w245:variant)
                n139 = Add(x=w227, y=w221) -> (x+y=w226:i32)
                n140 = call "Write Analog Variable Setups toIni.vi"("error in (no error)"=w273, "Path"=w246, "Enum with Variable List"=w248, "Analog User settigns"=w285, "Section(\"Default\")"=w235) -> ("error out"=w272:errorcluster)  [unwired: 10 in]
                n141 = Add(x=w225, y=w222) -> (x+y=w224:i32)
                n142 = call "Write Digital Variable Setups toIni.vi"("error in (no error)"=w272, "Path"=w246, "Enum with Variable List"=w245, "Digital User settigns"=w270, "Section(\"Default\")"=w236) -> ("error out"=w243:errorcluster)  [unwired: 10 in]
                n143 = Array Subset(array=w223, index=w226) -> (w230:T8[])  [unwired: 1 in]
                n144 = Array Subset(array=w229, index=w224) -> (w228:T20[])  [unwired: 1 in]
                n145 = call "GS Var Modem Status Common Ana User Settings.vi"("Action(GET)"=enum16{"GET", "SET"}."SET", "Modem Status analog var User settigns in"=w228, "Modem Status digital var User settigns in"=w230, "error in (no error)"=w243) -> ("error out"=w240:errorcluster)  [unwired: 9 in, 2 out]
                n146 = To Variant(anything=Variable_List_Modem_Status_Analog."TS_Signal_Quality" ("Variable ID")) -> (Variant=w232:variant)
                n147 = To Variant(anything=Variable_List_Modem_Status_Digital."TMU_LINK_STATUS" ("Enum")) -> (Variant=w231:variant)
                n148 = call "emi_Default Ini File Name.vi"("Name"="Modem Status Variables.ini" ("name or relative path")) -> ("Path"=w237:path)  [unwired: 13 in, 1 out]
                n149 = call "Write Analog Variable Setups toIni.vi"("error in (no error)"=w240, "Path"=w237, "Enum with Variable List"=w232, "Analog User settigns"=w228, "Section(\"Default\")"=w235) -> ("error out"=w241:errorcluster)  [unwired: 10 in]
                n150 = call "Write Digital Variable Setups toIni.vi"("error in (no error)"=w241, "Path"=w237, "Enum with Variable List"=w231, "Digital User settigns"=w230, "Section(\"Default\")"=w236) -> ("error out"=w239:errorcluster)  [unwired: 10 in]
                n151 = call "Normal User Default Chart holder FGV.vi"("Action(GET)"=T10."GET", "error in (no error)"=w239) -> ("Mem Ctl Out"=w261:T14, "error out"=w267:errorcluster)  [unwired: 12 in]
                n152 = Bundle By Name(cluster=w261, "UL1"="Upper left 1", "UL2"="Upper left 2", "UR1"="Upper right 1", "UR2"="Upper right 2", "LL1"="Lower left 1", "LL2"="Lower left 2", "LR1"="Lower right 1", "LR2"="Lower right 2") -> (w260:T14)
                n153 = call "Normal User Default Chart holder FGV.vi"("Action(GET)"=T10."SET", "Mem Ctl In"=w260, "error in (no error)"=w267) -> ("error out"=w265:errorcluster)  [unwired: 11 in, 1 out]
                n154 = call "Normal User Default Chart holder FGV.vi"("Action(GET)"=T10."Put in Ini", "error in (no error)"=w265) -> ("error out"=w266:errorcluster)  [unwired: 12 in, 1 out]
              }
            }
            n155 = call <vilib>:"Unset Busy.vi"("error in (no error)"=w216) -> ("error out"=w211:errorcluster)  [unwired: 10 in]
          }
          event "Cancel": Mouse Up {
            n156 = event-data() -> ()  [unwired: 1 in, 1 out]
          }
          event "List of Analog variables": Value Change {
            w298 = enum16{"GET", "SET"}."GET" ("Action(GET)")
            n157 = event-data() -> ("OldVal"=w336:i32, "NewVal"=w335:i32)  [unwired: 1 in]
            n158 = local read "User graph selection"() -> (w306:bool)
            n159 = local read "Unit"() -> (w302:u16)
            n160 = Bundle(cluster=T20 {"Scaling"={"Gain"=0.0, "Offset"=0.0}, "Limits and responces"={"Technical Error(NA)"={"Action"=enum."No Action", "Alarm"=FALSE}, "LL"={"Action"=enum."No Action", "Alarm"=FALSE}, "L"={"Action"=enum."No Action", "Alarm"=FALSE}, "H"={"Action"=enum."No Action", "Alarm"=FALSE}, "HH"={"Action"=enum."No Action", "Alarm"=FALSE}, "Limits"={"LL"=0.0, "L"=0.0, "H"=0.0, "HH"=0.0}}, "Allow Graph selection by user"=FALSE, "Unit"=0} ("element"), "Scaling"="Scaling", "Limits and responces"="Limits and responses", "Allow Graph selection by user"=w306, "Unit"=w302) -> (w327:T20)
            n161 = case shown="True" w316 {
              tunnel: [w340 w348] -> w310
              tunnel: w338 -> [w340 w348]
              tunnel: w337 -> [w342 w347]
              tunnel: [w342 w346] -> w330
              tunnel: w327 -> [_ w345]
              tunnel: w336 -> [_ w344]
              tunnel: w335 -> [w341 w343]
              tunnel: [w341 w343] -> w329
              frame False {
              }
              frame True {
                # "Super user"
                n162 = in-place {
                  in-place-border: w345 -> [w349]
                  n163 = in-place-array #3(w347, w344) -> ()  [unwired: 1 out]
                  n164 = in-place-array #3(w349) -> (w346:T20[])  [unwired: 1 out]
                }
              }
            }
            n165 = call "GS Var Common Ana Fixed Settings.vi"("Action(GET)"=w298, "error in (no error)"=w310) -> ("Common Analog Var Fixed out"=w307:T15[], "error out"=w309:errorcluster)  [unwired: 11 in, 1 out]
            n166 = call "GS Var TOOL Ana Fixed Settings.vi"("Action(GET)"=w298, "error in (no error)"=w309) -> ("Tool Analog var Fixed out"=w328:T15[], "error out"=w299:errorcluster)  [unwired: 11 in, 1 out]
            n167 = call "GS Var Modem Status Ana Fixed Settings.vi"("Action(GET)"=w298, "error in (no error)"=w299) -> ("Modem Status Analog var Fixed out"=w296:T15[], "error out"=w297:errorcluster)  [unwired: 11 in, 1 out]
            n168 = Build Array (concatenate)(w307, w328, w296) -> (w308:T15[])
            n169 = Index Array(array=w308, index=w329) -> (element=w334:T15)
            n170 = Index Array(array=w330, index=w329) -> (element=w321:T20)
            n171 = Unbundle By Name(w334) -> ("User adjustable Scaling"=w317:bool, "Comment"=→"Description":string, "Name"=→"Name":string, "Maximum upd"=→"Validity":T1, "Quantity"=w301:T16)
            n172 = Unbundle By Name(w321) -> ("Allow Graph selection by user"=w304:bool, "Scaling"=w323:T2, "Limits and responces"=w322:T3, "Unit"=w300:u16)
            n173 = And(x=w316, y=w317) -> (x .and. y?=w305:T12)
            n174 = local write "User graph selection"(w304) -> ()
            n175 = local write "Scaling"(w323) -> ()
            n176 = local write "Limits and responses"(w322) -> ()
            n177 = control-ref of="Scaling"() -> (w318:refnum<vi>)
            n178 = Select(t=T13."Enabled" ("Disabled"), s=w305, f=T13."Disabled and Grayed Out" ("Disabled")) -> (s? t:f=w315:T13)
            n179 = control-ref of="Unit"() -> (w303:refnum<vi>)
            n180 = property class="Clust (strict)"(reference=w318, error in=w297, "DisabledEnum"=w315) -> (reference out=w320:refnum<vi>, error out=w319:errorcluster)
            n181 = property on="Calibrate" class="Bool"("DisabledEnum"=w315) -> ()  [unwired: 2 in, 2 out]
            n182 = call "Initialize Unit Ring Control.vi"("Value"=w300, "Quantity"=w301, "Ctrl Ref"=w303) -> ()  [unwired: 9 in]
            n183 = Close Reference(reference=w320, error in (no error)=w319) -> (error out=w312:errorcluster)
          }
          event "Unit": Value Change {
            w351 = enum16{"GET", "SET"}."GET" ("Action(GET)")
            n184 = event-data() -> ("NewVal"=w354:u16, "OldVal"=w353:u16)  [unwired: 1 in]
            n185 = call "GS Var Common Ana Fixed Settings.vi"("Action(GET)"=w351) -> ("Common Analog Var Fixed out"=w359:T15[], "error out"=w361:errorcluster)  [unwired: 12 in, 1 out]
            n186 = call "GS Var TOOL Ana Fixed Settings.vi"("Action(GET)"=w351, "error in (no error)"=w361) -> ("Tool Analog var Fixed out"=w362:T15[], "error out"=w352:errorcluster)  [unwired: 11 in, 1 out]
            n187 = call "GS Var Modem Status Ana Fixed Settings.vi"("Action(GET)"=w351, "error in (no error)"=w352) -> ("Modem Status Analog var Fixed out"=w350:T15[])  [unwired: 11 in, 2 out]
            n188 = Build Array (concatenate)(w359, w362, w350) -> (w360:T15[])
            n189 = Index Array(array=w360, index=w357) -> (element=w363:T15)
            n190 = Unbundle By Name(w363) -> ("User adjustable Scaling"=w358:bool, "Quantity"=w356:T16)
            n191 = case shown="True" w358 {
              tunnel: w356 -> [w371 w379]
              tunnel: w354 -> [w370 w385]
              tunnel: w353 -> [_ w378]
              frame False {
                # "User adjustable scaling is not available\nuse only the unit conversion for scaling"
                n192 = call "Get Unit Scaling.vi"("Unit Index"=w370, "Quantity"=w371) -> ("Offset"=w367:dbl, "Gain"=w368:dbl)  [unwired: 7 in, 1 out]
                n193 = Bundle(cluster=T2 {"Gain"=1.0, "Offset"=0.0} ("Scaling"), "Gain"=w368, "Offset"=w367) -> (w366:T2)
                n194 = local write "Scaling"(w366) -> ()
              }
              frame True {
                # "apply new \nconversion"
                # "return to default\nscaling"
                # "If the variable is scalable by the user\nnew scaling values are calculated when\nthe unit changes."
                n195 = local read "Scaling"() -> (w384:T2)
                n196 = call "Get Unit Scaling.vi"("Unit Index"=w385, "Quantity"=w379) -> ("Offset"=w382:dbl, "Gain"=w383:dbl)  [unwired: 7 in, 1 out]
                n197 = call "Get Unit Scaling.vi"("Unit Index"=w378, "Quantity"=w379) -> ("Offset"=w376:dbl, "Gain"=w374:dbl)  [unwired: 7 in, 1 out]
                n198 = Unbundle(w384) -> ("Gain"=w375:dbl, "Offset"=w377:dbl)
                n199 = Subtract(x=w377, y=w376) -> (x-y=w372:dbl)
                n200 = Divide(x=w375, y=w374) -> (x/y=w373:dbl)
                n201 = Multiply(x=w383, y=w373) -> (x*y=w381:dbl)
                n202 = Add(x=w382, y=w372) -> (x+y=w380:dbl)
                n203 = Bundle(cluster=T2 {"Gain"=1.0, "Offset"=0.0} ("Scaling"), "Gain"=w381, "Offset"=w380) -> (w386:T2)
                n204 = local write "Scaling"(w386) -> ()
              }
            }
          }
          event "List of Digital variables": Value Change {
            w389 = enum16{"GET", "SET"}."GET" ("Action(GET)")
            n205 = event-data() -> ("OldVal"=w409:i32, "NewVal"=w407:i32)  [unwired: 1 in]
            n206 = case shown="True" w411 {
              tunnel: [w415 w422] -> w405
              tunnel: w412 -> [w415 w422]
              tunnel: w410 -> [w416 w421]
              tunnel: [w416 w420] -> w394
              tunnel: w409 -> [_ w419]
              tunnel: "User settings" -> [_ w418]
              tunnel: [w414 w417] -> w393
              tunnel: w407 -> [w414 w417]
              frame False {
              }
              frame True {
                n207 = in-place {
                  in-place-border: w418 -> [w423]
                  n208 = in-place-array #4(w421, w419) -> ()  [unwired: 1 out]
                  n209 = in-place-array #4(w423) -> (w420:T8[])  [unwired: 1 out]
                }
              }
            }
            n210 = call "GS Var Common Ana Fixed Settings.vi"("Action(GET)"=w389, "error in (no error)"=w405) -> ("Common Digital var Fixed"=w404:T19[], "error out"=w406:errorcluster)  [unwired: 11 in, 1 out]
            n211 = call "GS Var TOOL Ana Fixed Settings.vi"("Action(GET)"=w389, "error in (no error)"=w406) -> ("Tool Digital Var Fixed out"=w403:T19[], "error out"=w391:errorcluster)  [unwired: 11 in, 1 out]
            n212 = Index Array(array=w394, index=w393) -> (element=w392:T8)
            n213 = call "GS Var Modem Status Ana Fixed Settings.vi"("Action(GET)"=w389, "error in (no error)"=w391) -> ("Modem Status Digital Var Fixed out"=w388:T19[], "error out"=w390:errorcluster)  [unwired: 11 in, 1 out]
            n214 = local write "User settings"(w392) -> ()
            n215 = Build Array (concatenate)(w404, w403, w388) -> (w402:T19[])
            n216 = Index Array(array=w402, index=w393) -> (element=w401:T19)
            n217 = Unbundle By Name(w401) -> ("Comment"=→"Description Dig":string, "Name"=→"Name Dig":string, "Maximum upd"=→"Validity Dig":T1, "On Text"=→"On indication":string, "Off Text"=→"Off Indication":string, "NA Text"=→"NA Indicatino":string)
          }
          event "Help": Value Change {
            n218 = event-data() -> ()  [unwired: 1 in, 1 out]
            n219 = case shown="True" "Help" {
              tunnel: [w431 w433] -> w429
              tunnel: w428 -> [w431 w432]
              tunnel: w425 -> [_ _]
              frame False {
              }
              frame True {
                n220 = call "Open App Help file.vi"("error In"=w432) -> ("error out"=w433:errorcluster)  [unwired: 14 in]
              }
            }
          }
          event "Calibrate": Value Change {
            n221 = event-data() -> ()  [unwired: 1 in, 1 out]
            n222 = property on="List of Analog variables" class="LstBox (strict)"() -> ("Item Names"=w438:string[])  [unwired: 2 in, 2 out]
            n223 = Index Array(array=w438, index=w437) -> (element=w436:string)
            n224 = local read "Scaling"() -> (w435:T2)
            n225 = Unbundle By Name(w435) -> ("Gain"=w434:dbl)
            n226 = call "Channel Calibration.vi"("error in (no error)"=w446, "Gain"=w434, "Channel Name"=w436, "index"=w437) -> ("error out"=w445:errorcluster, "Offset"=w439:dbl, "Gain"=w440:dbl, "Status Output"=w444:T27)  [unwired: 4 in]
            n227 = Unbundle By Name(w444) -> ("Keep"=w443:bool, "Zero"=w442:bool, "2 point"=w441:bool)
            n228 = case shown="True" w443 {
              tunnel: w442 -> [_ w453]
              tunnel: w441 -> [_ w450]
              tunnel: w440 -> [_ w449]
              tunnel: w439 -> [_ w452]
              frame False {
              }
              frame True {
                n229 = case shown="False" w453 {
                  tunnel: w452 -> [w454 w464]
                  tunnel: [w456 w463] -> w451
                  tunnel: w450 -> [w457 _]
                  tunnel: w449 -> [w455 _]
                  frame False {
                    n230 = case shown="True" w457 {
                      tunnel: [w458 w461] -> w456
                      tunnel: w455 -> [_ w460]
                      tunnel: w454 -> [_ w459]
                      frame False {
                        n231 = local read "Scaling"() -> (w458:T2)
                      }
                      frame True {
                        n232 = Bundle By Name(cluster=T2 {"Gain"=1.0, "Offset"=0.0} ("output cluster"), "Gain"=w460, "Offset"=w459) -> (w461:T2)
                      }
                    }
                  }
                  frame True {
                    n233 = local read "Scaling"() -> (w465:T2)
                    n234 = Bundle By Name(cluster=w465, "Offset"=w464) -> (w463:T2)
                  }
                }
                n235 = local write "Scaling"(w451) -> ()
              }
            }
          }
        }
      }
    }
    frame Error {
      n236 = Unbundle(w471) -> ("code"=w468:i32, "source"=w467:string)  [unwired: 1 out]
      n237 = Format Into String(format string="%d    %s", initial string="Options dialog could not be displayed due to error\n\n" ("message"), w468, w467) -> (resulting string=w469:string)  [unwired: 1 in, 1 out]
      n238 = One Button Dialog(message=w469) -> ()  [unwired: 1 in, 1 out]
    }
  }
  "OK" <- w17
  n239 = call "emi_Dialog End.vi"("error in"=w16) -> ("error out"=→"error out":errorcluster)  [unwired: 14 in]
